vi "Get settings chain.vi"(8 "error in (no error)":errorcluster, 11 "WaveformBase in":refnum<class "Waveform.lvclass">) -> (0 "error out":errorcluster, 1 "class name":string[](array[string]), 2 "settings":variant[](array[variant]), 3 "WaveformBase out":refnum<class "Waveform.lvclass">)   [LabVIEW 2012, in "Waveform.lvclass"]
doc: "Returns an array of variants containing the settings clusters of each class in the inheritance chain (lowest child class first), together with an array of all class names in the inheritance chain.\n\nFor classes without settings cluster, the settings chain contains empty variants."
uses:
  Waveform.lvclass
  <vilib>/Distrio/Murmex/Murmex/Murmex.lvclass
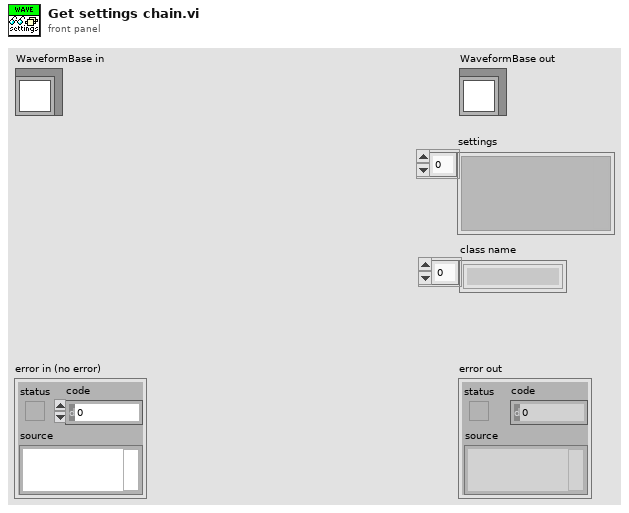
[diagram p1: front panel]
types:
  T1 = typedef "Waveform.lvclass/settings.ctl" = cluster{"counter_set":T2, "AO_set":T3, "Pockels Cell":T5}
  T2 = typedef "Waveform.lvclass/counter_set.ctl" = cluster{"Numeric":dbl}
  T3 = typedef "Waveform.lvclass/AO_set.ctl" = cluster{"Orca":cluster{"HSYNC":dbl, "frame_rate":dbl, "y_res":dbl, "line_exp":dbl[unit], "rolling_shutter":dbl[unit]}, "waveform data 1":T4, "waveform data 2":T4}
  T4 = typedef "Waveform.lvclass/waveform data.ctl" = cluster{"amplitude":dbl[unit], "offset":dbl[unit], "delay":dbl[unit], "duty cycle":dbl, "sampling info":cluster{"Fs":dbl, "#s":dbl}, "frequency":dbl[unit], "phase":dbl[unit]}
  T5 = typedef "Waveform.lvclass/pockels cell.ctl" = cluster{"digital ratio":dbl, "pulses per pixel":dbl, "Wavelength":T6}
  T6 = typedef "Waveform.lvclass/wavelength.ctl" = dbl
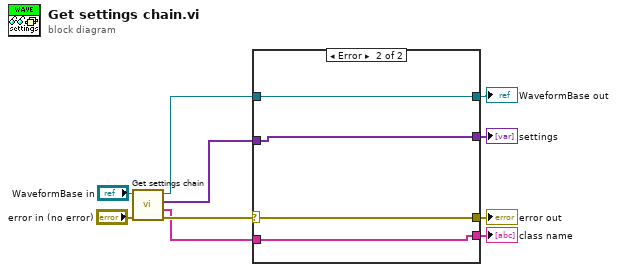
[diagram p0: block diagram]
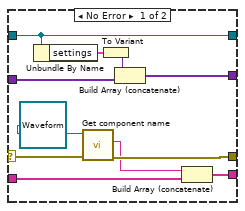
[diagram p2: hidden frame]
diagram:
  n1 = call-parent "Get settings chain.vi"("error in (no error)"="error in (no error)", "MurmexBase in"="WaveformBase in") -> ("error out"=w8:errorcluster, "class name"=w4:string[], "settings"=w1:variant[], "MurmexBase out"=w6:refnum<class "Waveform.lvclass">)  [unwired: 6 in]
  n2 = case shown="Error" w8 {
    selector: w8 -> [w21 w25]
    tunnel: [w20 w25] -> w7
    tunnel: w6 -> [w13 w24]
    tunnel: [w13 w24] -> w5
    tunnel: w4 -> [w16 w22]
    tunnel: [w14 w22] -> w3
    tunnel: [w12 w23] -> w2
    tunnel: w1 -> [w11 w23]
    frame No Error {
      n3 = Unbundle By Name(w13) -> ("settings"=w18:T1)
      n4 = call <vilib>:"Get component name.vi"("error in (no error)"=w21, "Murmex in"=refnum<class "Waveform.lvclass"> refnum ("Waveform")) -> ("error out"=w20:errorcluster, "component name"=w15:string)  [unwired: 7 in, 1 out]
      n5 = To Variant(anything=w18) -> (Variant=w19:variant)
      n6 = Build Array (concatenate)(w19, w11) -> (w12:variant[])
      n7 = Build Array (concatenate)(w15, w16) -> (w14:string[])
    }
    frame Error {
    }
  }
  "error out" <- w7
  "WaveformBase out" <- w5
  "settings" <- w2
  "class name" <- w3
